vi "RichToFlatcif_plugincore_GetStatusDataResponse.vi"(5 "OutputClusterType":T1, 11 "InputCluster":T11) -> (3 "OutputCluster":T1)   [LabVIEW 2021, in "CIFCorePlugin_server.lvlib"]
uses:
  CIFCorePlugin_server.lvlib
  cif_plugincore_GetStatusDataResponse.ctl
  cif_management_common_PluginStatusData.ctl
  cif_management_common_PluginStatusData_PluginState.ctl
  cif_management_common_TimingStatistics.ctl
  cif_common_TimingStats.ctl
  cif_management_common_FifoStatistics.ctl
  cif_management_common_Error.ctl
  cif_management_common_MonitorDoubles.ctl
  cif_management_common_MonitorU64.ctl
  cif_management_common_MonitorI64.ctl
  cif_plugincore_GetStatusDataResponse_Flat.ctl
  cif_management_common_PluginStatusData_Flat.ctl
  cif_management_common_TimingStatistics_Flat.ctl
  cif_common_TimingStats_Flat.ctl
  cif_management_common_FifoStatistics_Flat.ctl
  cif_management_common_Error_Flat.ctl
  cif_management_common_MonitorDoubles_Flat.ctl
  cif_management_common_MonitorU64_Flat.ctl
  cif_management_common_MonitorI64_Flat.ctl
  RichToFlatcif_management_common_TimingStatistics.vi
  RichToFlatcif_management_common_FifoStatistics.vi
  RichToFlatcif_management_common_Error.vi
  RichToFlatcif_management_common_MonitorDoubles.vi
  RichToFlatcif_management_common_MonitorU64.vi
  RichToFlatcif_management_common_MonitorI64.vi
  RichToFlatcif_common_TimingStats.vi
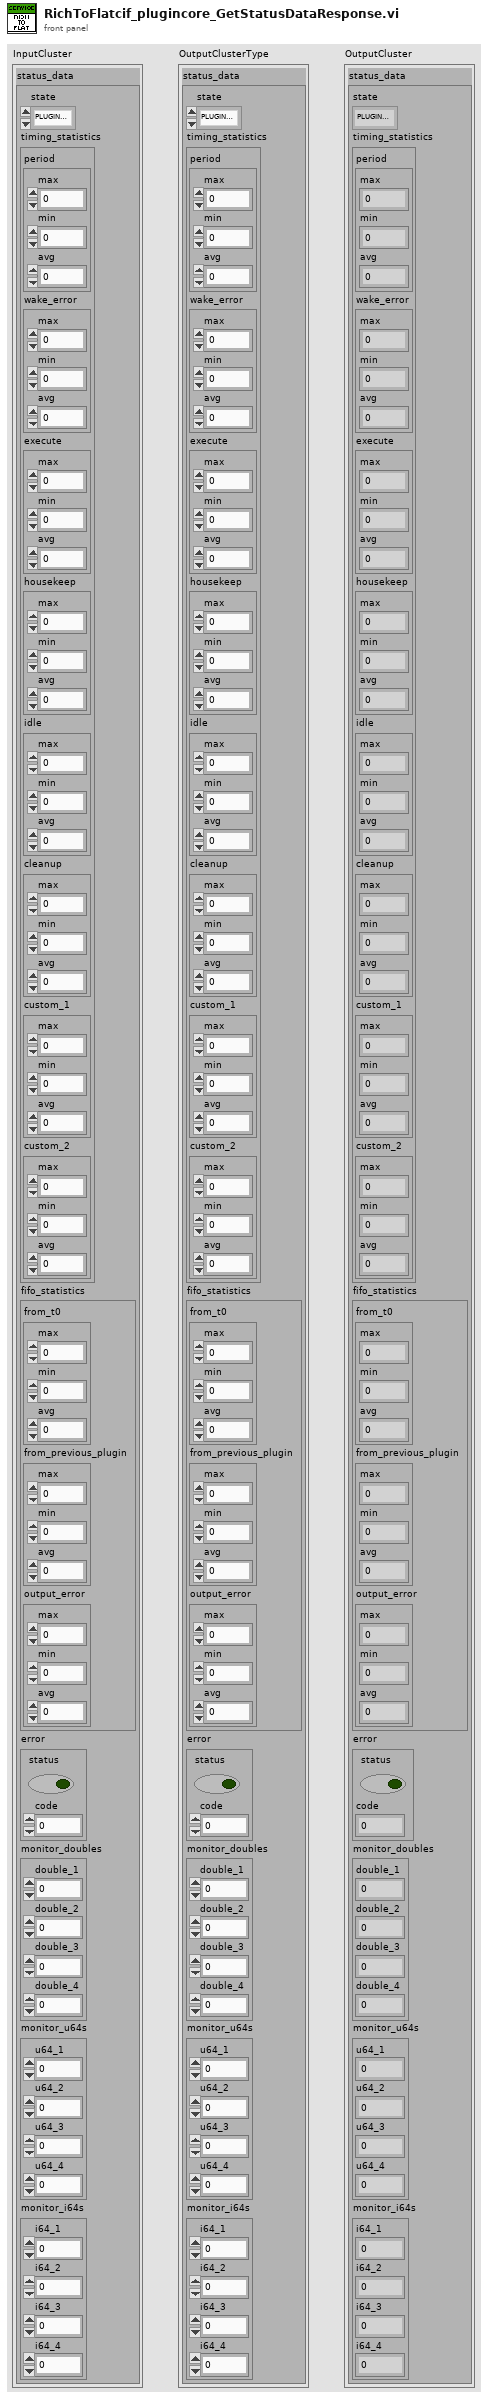
[diagram p1: front panel]
types:
  T1 = typedef "CIFCorePlugin_server.lvlib/cif_plugincore_GetStatusDataResponse_Flat.ctl" = cluster{"status_data":T2}
  T2 = typedef "CIFCorePlugin_server.lvlib/cif_management_common_PluginStatusData_Flat.ctl" = cluster{"state":T3, "timing_statistics":T4, "fifo_statistics":T6, "error":T7, "monitor_doubles":T8, "monitor_u64s":T9, "monitor_i64s":T10}
  T3 = typedef "CIFCorePlugin_server.lvlib/cif_management_common_PluginStatusData_PluginState.ctl" = enum32{"PLUGINSTATE_UNKNOWN", "PLUGINSTATE_CREATING", "PLUGINSTATE_LISTENING", "PLUGINSTATE_RUNNING", "PLUGINSTATE_CLEANINGUP", "PLUGINSTATE_DESTROYING"}
  T4 = typedef "CIFCorePlugin_server.lvlib/cif_management_common_TimingStatistics_Flat.ctl" = cluster{"period":T5, "wake_error":T5, "execute":T5, "housekeep":T5, "idle":T5, "cleanup":T5, "custom_1":T5, "custom_2":T5}
  T5 = typedef "CIFCorePlugin_server.lvlib/cif_common_TimingStats_Flat.ctl" = cluster{"max":i64, "min":i64, "avg":dbl}
  T6 = typedef "CIFCorePlugin_server.lvlib/cif_management_common_FifoStatistics_Flat.ctl" = cluster{"from_t0":T5, "from_previous_plugin":T5, "output_error":T5}
  T7 = typedef "CIFCorePlugin_server.lvlib/cif_management_common_Error_Flat.ctl" = cluster{"status":bool, "code":i32}
  T8 = typedef "CIFCorePlugin_server.lvlib/cif_management_common_MonitorDoubles_Flat.ctl" = cluster{"double_1":dbl, "double_2":dbl, "double_3":dbl, "double_4":dbl}
  T9 = typedef "CIFCorePlugin_server.lvlib/cif_management_common_MonitorU64_Flat.ctl" = cluster{"u64_1":u64, "u64_2":u64, "u64_3":u64, "u64_4":u64}
  T10 = typedef "CIFCorePlugin_server.lvlib/cif_management_common_MonitorI64_Flat.ctl" = cluster{"i64_1":i64, "i64_2":i64, "i64_3":i64, "i64_4":i64}
  T11 = typedef "CIFCorePlugin_server.lvlib/cif_plugincore_GetStatusDataResponse.ctl" = cluster{"status_data":T12}
  T12 = typedef "CIFCorePlugin_server.lvlib/cif_management_common_PluginStatusData.ctl" = cluster{"state":T3, "timing_statistics":T13, "fifo_statistics":T15, "error":T16, "monitor_doubles":T17, "monitor_u64s":T18, "monitor_i64s":T19}
  T13 = typedef "CIFCorePlugin_server.lvlib/cif_management_common_TimingStatistics.ctl" = cluster{"period":T14, "wake_error":T14, "execute":T14, "housekeep":T14, "idle":T14, "cleanup":T14, "custom_1":T14, "custom_2":T14}
  T14 = typedef "CIFCorePlugin_server.lvlib/cif_common_TimingStats.ctl" = cluster{"max":i64, "min":i64, "avg":dbl}
  T15 = typedef "CIFCorePlugin_server.lvlib/cif_management_common_FifoStatistics.ctl" = cluster{"from_t0":T14, "from_previous_plugin":T14, "output_error":T14}
  T16 = typedef "CIFCorePlugin_server.lvlib/cif_management_common_Error.ctl" = cluster{"status":bool, "code":i32}
  T17 = typedef "CIFCorePlugin_server.lvlib/cif_management_common_MonitorDoubles.ctl" = cluster{"double_1":dbl, "double_2":dbl, "double_3":dbl, "double_4":dbl}
  T18 = typedef "CIFCorePlugin_server.lvlib/cif_management_common_MonitorU64.ctl" = cluster{"u64_1":u64, "u64_2":u64, "u64_3":u64, "u64_4":u64}
  T19 = typedef "CIFCorePlugin_server.lvlib/cif_management_common_MonitorI64.ctl" = cluster{"i64_1":i64, "i64_2":i64, "i64_3":i64, "i64_4":i64}
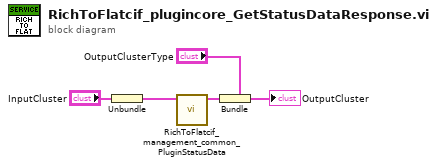
[diagram p0: block diagram]
diagram:
  n1 = Unbundle "Unbundle"("InputCluster") -> ("status_data"=w2:T12)
  n2 = call "RichToFlatcif_management_common_PluginStatusData.vi"("InputCluster"=w2) -> ("OutputCluster"=w1:T2)  [unwired: 10 in]
  n3 = Bundle "Bundle"(cluster="OutputClusterType", "status_data"=w1) -> (→"OutputCluster":T1)
